vi "mxwScript_API_XMLMakeDropRelationText.vi"(9 "addWireSpace":bool=TRUE, 10 "distance":i32 min=0, 11 "direction":T1) -> (3 "XML out":string)   [LabVIEW 2017]
uses:
  codeGenAPISupport.llb/cgAPI_mxwScript_DrpTmplt_SimpleDirection.ctl
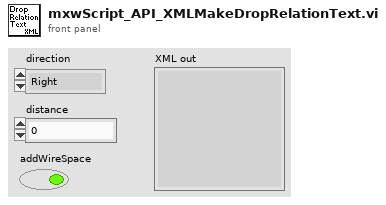
[diagram p1: front panel]
types:
  T1 = typedef "cgAPI_mxwScript_DrpTmplt_SimpleDirection.ctl" = enum16{"Right", "Left", "Below", "Above"}
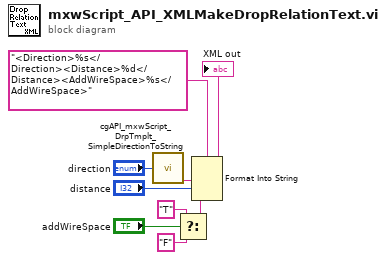
[diagram p0: block diagram]
diagram:
  n1 = call "cgAPI_mxwScript_DrpTmplt_SimpleDirectionToString.vi"("direction"="direction") -> ("string"=w2:string)  [unwired: 4 out]
  n2 = Select(t="T", s="addWireSpace", f="F") -> (s? t:f=w8:string)
  n3 = Format Into String(format string="<Direction>%s</Direction><Distance>%d</Distance><AddWireSpace>%s</AddWireSpace>", w2, "distance", w8) -> (resulting string=→"XML out":string)  [unwired: 2 in, 1 out]
